vi "InsertIntoArray_v2.vi"(0 "ROSCO Params":T2, 1 "KeyVal":T1, 3 "error in (no error)":errorcluster) -> (7 "ROSCO Params Out":T2, 10 "error out":errorcluster)   [LabVIEW 2018]
uses:
  Clusters/RoscoParams.ctl
  Clusters/SwapArrayCluster.ctl
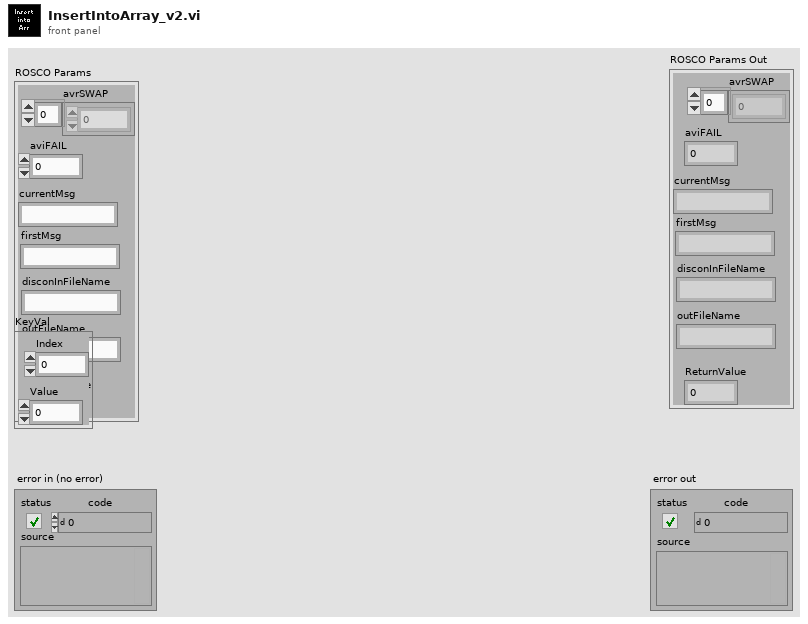
[diagram p1: front panel]
types:
  T1 = typedef "SwapArrayCluster.ctl" = cluster{"Index":i32, "Value":dbl}
  T2 = typedef "RoscoParams.ctl" = cluster{"avrSWAP":sgl[], "aviFAIL":i32, "currentMsg":string, "ReturnValue":i32, "disconInFileName":string, "outFileName":string, "firstMsg":string}
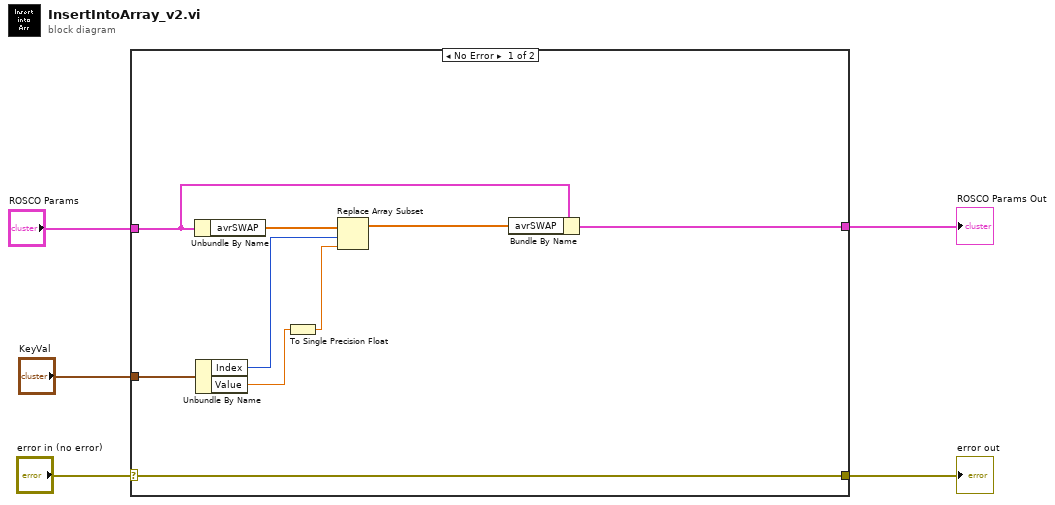
[diagram p0: block diagram]
diagram:
  n1 = case shown="No Error" "error in (no error)" {
    selector: "error in (no error)" -> [w14 w15]
    tunnel: "ROSCO Params" -> [w11 w16]
    tunnel: [w14 w15] -> w3
    tunnel: [w9 w16] -> w2
    tunnel: "KeyVal" -> [w8 _]
    frame No Error {
      n2 = Unbundle By Name(w11) -> ("avrSWAP"=w13:sgl[])
      n3 = Unbundle By Name(w8) -> ("Index"=w7:i32, "Value"=w6:dbl)
      n4 = To Single Precision Float(number=w6) -> (single precision float=w12:sgl)
      n5 = Replace Array Subset(array=w13, new element=w12, index=w7) -> (w10:sgl[])
      n6 = Bundle By Name(cluster=w11, "avrSWAP"=w10) -> (w9:T2)
    }
    frame Error {
    }
  }
  "error out" <- w3
  "ROSCO Params Out" <- w2
